vi "Compare Labels.vi"(9 "refresh listbox":T6[](array[typedef]), 10 "new label":T1, 11 "old label":T1) -> (1 "refresh listbox out":T6[](array[typedef]), 2 "any changes?":bool)   [LabVIEW 2024, in "AIM ARINC 429 System Explorer.lvlib" / "Implementation.lvlib"]
uses:
  Implementation.lvlib
  Types/Refresh Listbox.ctl
  Types/Refresh Symbols.ctl
  Shared/VS Channels Definition for Label.ctl
  Shared/VS Channel Definition for Parameter.ctl
  Shared/Parameter Definition.ctl
  <vilib>/NI/NI VeriStand Encoding and Decoding/Encoding.ctl
  Shared/Transfer Type.ctl
  Refresh Constants.vi
  <vilib>/NI/NI VeriStand Encoding and Decoding/Encoding and Decoding.lvlib
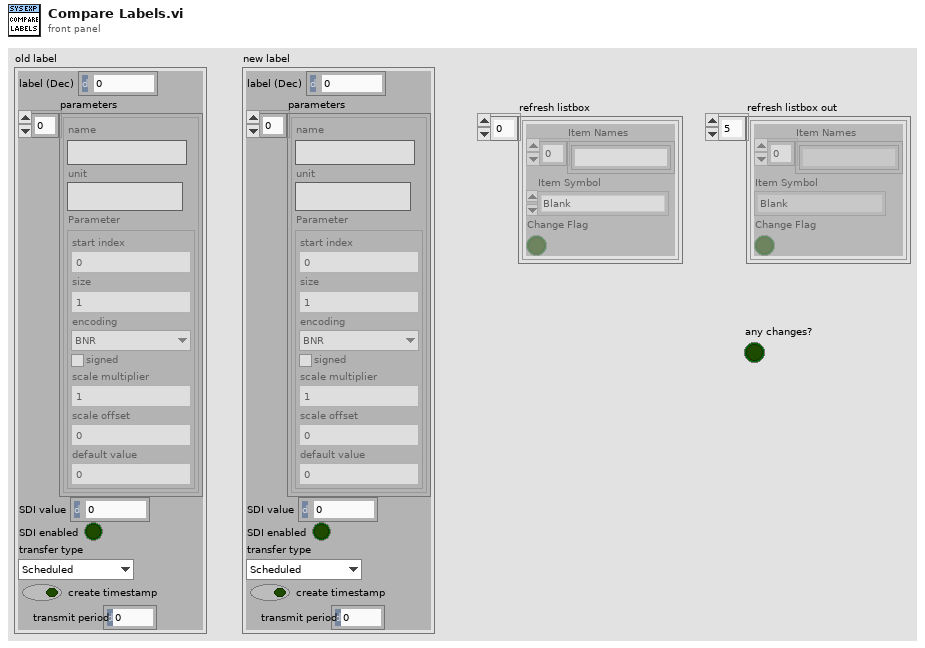
[diagram p1: front panel]
types:
  T1 = typedef "VS Channels Definition for Label.ctl" = cluster{"label (Dec)":u32, "parameters":T2[], "SDI value":u8, "SDI enabled":bool, "transfer type":T5, "create timestamp":bool, "transmit period":u32}
  T2 = typedef "VS Channel Definition for Parameter.ctl" = cluster{"name":string, "unit":string, "Parameter":T3}
  T3 = typedef "Parameter Definition.ctl" = cluster{"start index":i32, "size":i32, "encoding":T4, "signed":bool, "scale multiplier":dbl, "scale offset":dbl, "default value":dbl}
  T4 = typedef "Encoding and Decoding.lvlib/Encoding.ctl" = enum16{"BNR", "BCD", "Discrete"}
  T5 = typedef "Transfer Type.ctl" = enum16{"Scheduled", "Acyclic", "Block", "Strobe"}
  T6 = typedef "AIM ARINC 429 System Explorer.lvlib/Implementation.lvlib/Refresh Listbox.ctl" = cluster{"Item Names":string[], "Item Symbol":T7, "Change Flag":bool}
  T7 = typedef "AIM ARINC 429 System Explorer.lvlib/Implementation.lvlib/Refresh Symbols.ctl" = enum16{"Blank", "Port", "Incoming", "Outgoing", "Label", "Word", "Parameter", "ARINC-429", "Config Files", "Channel Spec", "Item"}
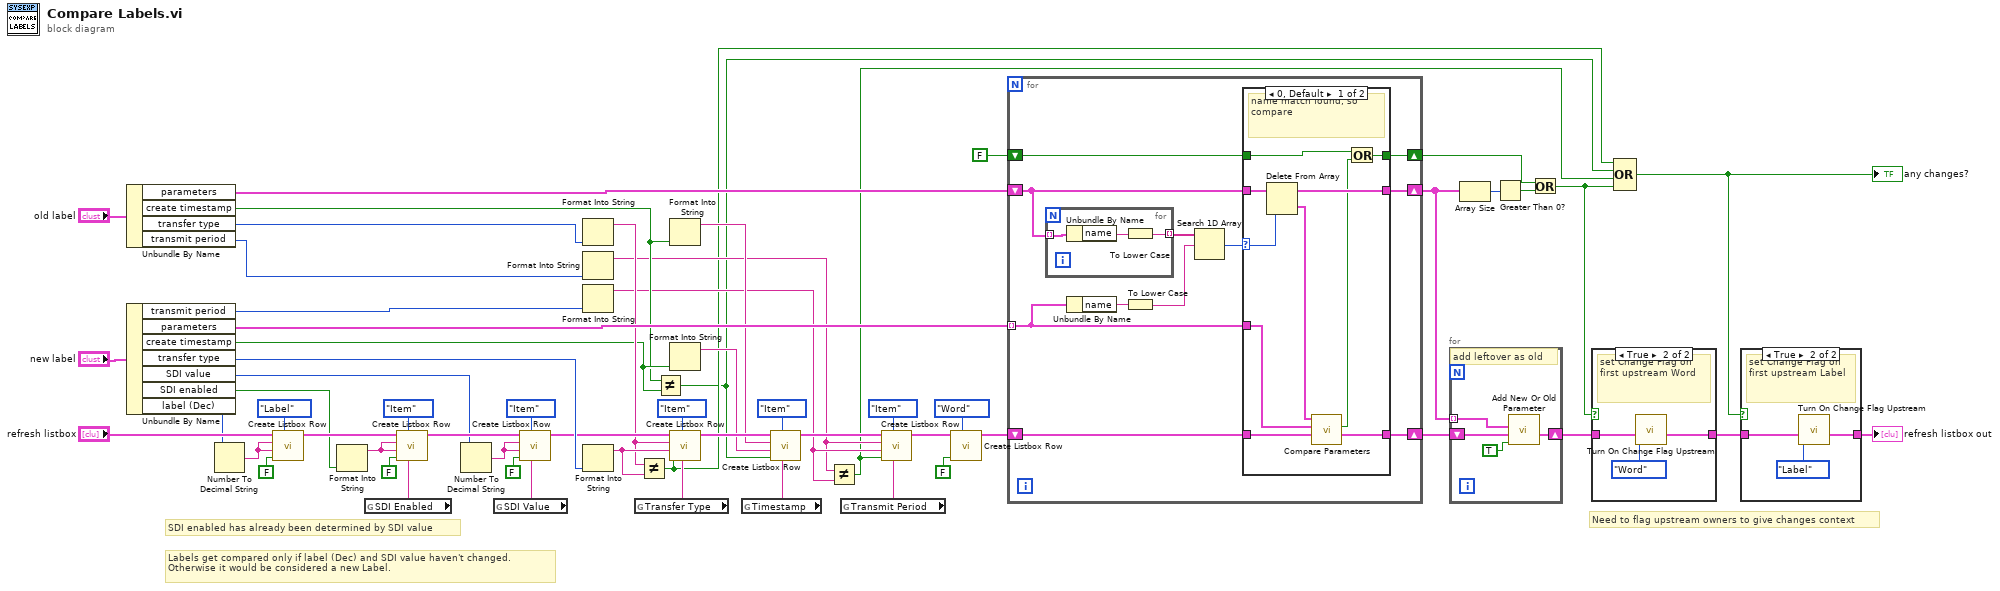
[diagram p0: block diagram]
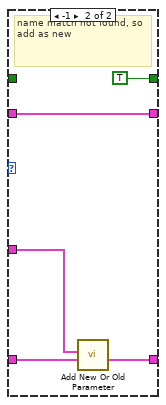
[diagram p4: hidden frame]
diagram:
  # "Labels get compared only if label (Dec) and SDI value haven't changed. Otherwise it would be considered a new Label."
  # "Need to flag upstream owners to give changes context"
  # "SDI enabled has already been determined by SDI value"
  n1 = Unbundle By Name("old label") -> ("parameters"=w37:T2[], "create timestamp"=w13:bool, "transfer type"=w41:T5, "transmit period"=w9:u32)
  n2 = Unbundle By Name("new label") -> ("transmit period"=w8:u32, "parameters"=w49:T2[], "create timestamp"=w14:bool, "transfer type"=w51:T5, "SDI value"=w54:u8, "SDI enabled"=w31:bool, "label (Dec)"=w58:u32)
  n3 = Number To Decimal String(number=w58) -> (decimal integer string=w44:string)  [unwired: 1 in]
  n4 = call "Create Listbox Row.vi"("refresh symbol (Blank)"=Refresh_Symbols."Label" ("Refresh Symbol (Blank)"), "change? (T)"=FALSE, "new item"=w44, "old item"=w44, "refresh listbox"="refresh listbox") -> ("refresh listbox out"=w56:T6[])  [unwired: 6 in]
  n5 = Format Into String(w31) -> (resulting string=w20:string)  [unwired: 3 in, 1 out]
  n6 = global read "Refresh Constants.vi" "SDI Enabled"() -> (w35:string)
  n7 = call "Create Listbox Row.vi"("override name"=w35, "refresh symbol (Blank)"=Refresh_Symbols."Item" ("Refresh Symbol (Blank)"), "change? (T)"=FALSE, "new item"=w20, "old item"=w20, "refresh listbox"=w56) -> ("refresh listbox out"=w55:T6[])  [unwired: 5 in]
  n8 = Number To Decimal String(number=w54) -> (decimal integer string=w42:string)  [unwired: 1 in]
  n9 = global read "Refresh Constants.vi" "SDI Value"() -> (w33:string)
  n10 = call "Create Listbox Row.vi"("override name"=w33, "refresh symbol (Blank)"=Refresh_Symbols."Item" ("Refresh Symbol (Blank)"), "change? (T)"=FALSE, "new item"=w42, "old item"=w42, "refresh listbox"=w55) -> ("refresh listbox out"=w50:T6[])  [unwired: 5 in]
  n11 = Format Into String(w41) -> (resulting string=w38:string)  [unwired: 3 in, 1 out]
  n12 = Format Into String(w9) -> (resulting string=w5:string)  [unwired: 3 in, 1 out]
  n13 = Format Into String(w8) -> (resulting string=w6:string)  [unwired: 3 in, 1 out]
  n14 = Format Into String(w51) -> (resulting string=w39:string)  [unwired: 3 in, 1 out]
  n15 = global read "Refresh Constants.vi" "Transfer Type"() -> (w34:string)
  n16 = Not Equal?(x=w38, y=w39) -> (x != y?=w3:bool)
  n17 = Not Equal?(x=w13, y=w14) -> (x != y?=w2:bool)
  n18 = Format Into String(w13) -> (resulting string=w16:string)  [unwired: 3 in, 1 out]
  n19 = Format Into String(w14) -> (resulting string=w15:string)  [unwired: 3 in, 1 out]
  n20 = call "Create Listbox Row.vi"("override name"=w34, "refresh symbol (Blank)"=Refresh_Symbols."Item" ("Refresh Symbol (Blank)"), "change? (T)"=w3, "new item"=w39, "old item"=w38, "refresh listbox"=w50) -> ("refresh listbox out"=w17:T6[])  [unwired: 5 in]
  n21 = global read "Refresh Constants.vi" "Timestamp"() -> (w12:string)
  n22 = call "Create Listbox Row.vi"("override name"=w12, "refresh symbol (Blank)"=Refresh_Symbols."Item" ("Refresh Symbol (Blank)"), "change? (T)"=w2, "new item"=w15, "old item"=w16, "refresh listbox"=w17) -> ("refresh listbox out"=w10:T6[])  [unwired: 5 in]
  n23 = Not Equal?(x=w5, y=w6) -> (x != y?=w1:bool)
  n24 = global read "Refresh Constants.vi" "Transmit Period"() -> (w4:string)
  n25 = call "Create Listbox Row.vi"("override name"=w4, "refresh symbol (Blank)"=Refresh_Symbols."Item" ("Refresh Symbol (Blank)"), "change? (T)"=w1, "new item"=w6, "old item"=w5, "refresh listbox"=w10) -> ("refresh listbox out"=w7:T6[])  [unwired: 5 in]
  n26 = call "Create Listbox Row.vi"("refresh symbol (Blank)"=Refresh_Symbols."Word" ("Refresh Symbol (Blank)"), "change? (T)"=FALSE, "refresh listbox"=w7) -> ("refresh listbox out"=w47:T6[])  [unwired: 8 in]
  n27 = for {
    shift-right: [w70] -> w32
    shift-left: w47 -> [w71]
    tunnel: w49 -> [w69] mode=indexing
    shift-right: [w63] -> w29
    shift-left: w37 -> [w64]
    shift-right: [w61] -> w26
    shift-left: FALSE -> [w62]
    n28 = for {
      tunnel: w64 -> [w88] mode=indexing
      tunnel: [w87] -> w67 mode=indexing
      n29 = Unbundle By Name(w88) -> ("name"=w89:string)
      n30 = To Lower Case(string=w89) -> (all lower case string=w87:string)
    }
    n31 = Unbundle By Name(w69) -> ("name"=w68:string)
    n32 = To Lower Case(string=w68) -> (all lower case string=w66:string)
    n33 = Search 1D Array(1D array=w67, element=w66) -> (index of element=w65:i32)  [unwired: 1 in]
    n34 = case shown="0, Default" w65 {
      selector: w65 -> [w80 _]
      tunnel: w71 -> [w77 w86]
      tunnel: [w78 w84] -> w70
      tunnel: w69 -> [w76 w85]
      tunnel: [w79 w83] -> w63
      tunnel: w64 -> [w81 w83]
      tunnel: w62 -> [w73 _]
      tunnel: [w74 TRUE] -> w61
      frame 0, Default {
        # "name match found, so compare"
        n35 = Delete From Array(array=w81, index=w80) -> (deleted portion=w75:T2, array with subset deleted=w79:T2[])  [unwired: 1 in]
        n36 = call "Compare Parameters.vi"("refresh listbox"=w77, "new parameter"=w76, "old parameter"=w75) -> ("refresh listbox out"=w78:T6[], "any changes?"=w72:bool)  [unwired: 7 in]
        n37 = Or(x=w73, y=w72) -> (x .or. y?=w74:bool)
      }
      frame -1 {
        # "name match not found, so add as new"
        n38 = call "Add New Or Old Parameter.vi"("refresh listbox"=w86, "channel parameter"=w85) -> ("refresh listbox out"=w84:T6[])  [unwired: 9 in]
      }
    }
  }
  n39 = for {
    shift-right: [w91] -> w25
    shift-left: w32 -> [w93]
    tunnel: w29 -> [w90] mode=indexing
    # "add leftover as old"
    n40 = call "Add New Or Old Parameter.vi"("old port?"=TRUE, "refresh listbox"=w93, "channel parameter"=w90) -> ("refresh listbox out"=w91:T6[])  [unwired: 8 in]
  }
  n41 = Array Size(array=w29) -> (size(s)=w28:i32)
  n42 = Greater Than 0?(x=w28) -> (x > 0?=w27:bool)
  n43 = Or(x=w26, y=w27) -> (x .or. y?=w24:bool)
  n44 = case shown="True" w24 {
    tunnel: w25 -> [w94 w97]
    tunnel: [w94 w95] -> w23
    frame False {
    }
    frame True {
      # "set Change Flag on first upstream Word"
      n45 = call "Turn On Change Flag Upstream.vi"("symbol to change"=Refresh_Symbols."Word", "refresh listbox"=w97) -> ("refresh listbox out"=w95:T6[])  [unwired: 9 in]
    }
  }
  n46 = Compound Arithmetic op=OR(w3, w2, w1, w24) -> (w22:bool)
  "any changes?" <- w22
  n47 = case shown="True" w22 {
    tunnel: w23 -> [w98 w99]
    tunnel: [w98 w100] -> w21
    frame False {
    }
    frame True {
      # "set Change Flag on first upstream Label"
      n48 = call "Turn On Change Flag Upstream.vi"("symbol to change"=Refresh_Symbols."Label", "refresh listbox"=w99) -> ("refresh listbox out"=w100:T6[])  [unwired: 9 in]
    }
  }
  "refresh listbox out" <- w21
